vi "build_path.vi"(7 "filepath":path, 10 "path":string, 11 "base_path":string) -> (3 "path":string)   [LabVIEW 2015, in "lv-dropbox.lvlib"]
uses:
  lv-dropbox.lvlib
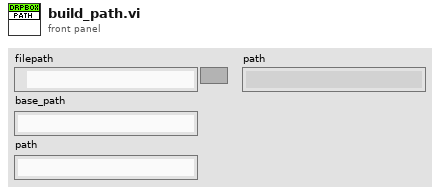
[diagram p1: front panel]
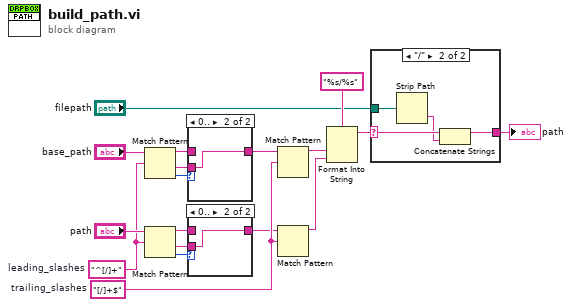
[diagram p0: block diagram]
diagram:
  w15 = "^[/]+"  # leading_slashes
  w14 = "[/]+$"  # trailing_slashes
  n1 = Match Pattern(string="base_path", regular expression=w15) -> (before substring=w11:string, after substring=w10:string, offset past match=w8:i32)  [unwired: 1 in, 1 out]
  n2 = Match Pattern(string="path", regular expression=w15) -> (before substring=w5:string, after substring=w6:string, offset past match=w7:i32)  [unwired: 1 in, 1 out]
  n3 = case shown="0.." w8 {
    tunnel: w11 -> [w19 _]
    tunnel: w10 -> [_ w20]
    tunnel: [w19 w20] -> w9
    frame Default {
    }
    frame 0.. {
    }
  }
  n4 = case shown="0.." w7 {
    tunnel: w5 -> [w21 _]
    tunnel: w6 -> [_ w22]
    tunnel: [w21 w22] -> w4
    frame Default {
    }
    frame 0.. {
    }
  }
  n5 = Match Pattern(string=w9, regular expression=w14) -> (before substring=w13:string)  [unwired: 1 in, 3 out]
  n6 = Match Pattern(string=w4, regular expression=w14) -> (before substring=w12:string)  [unwired: 1 in, 3 out]
  n7 = Format Into String(format string="%s/%s", w13, w12) -> (resulting string=w2:string)  [unwired: 2 in, 1 out]
  n8 = case shown="\"/\"" w2 {
    selector: w2 -> [w23 w26]
    tunnel: "filepath" -> [_ w27]
    tunnel: [w23 w25] -> w1
    frame Default {
    }
    frame "/" {
      n9 = Strip Path(path=w27) -> (name=w24:string)  [unwired: 1 out]
      n10 = Concatenate Strings(w26, w24) -> (w25:string)
    }
  }
  "path" <- w1
